vi "get_goal_filter.vi"(4 "Parameters":T2={"Stimulus"={"Type"=enum."Off", "Phase"=0.0, "Amplitude"=[], "Injection point"=enum."Total pose", "Closed loop"=FALSE, "Offset"=[], "Tip -> world"=FALSE, "Frequency"=0.0, "Length"=0.0}, "Goal Filter A"={"Speedup max"=0.0, "Speedup thresh"=0.0, "Speedup nonlin"=0.0, "Filters"=[]}, "Mode controls"={"Hold"=FALSE, "Cancellation"=FALSE, "Goal filter"=FALSE, "Trigger"=FALSE}, "Manipulator type"=enum."Current piezo", "Manipulator calibration"={"Tool offsets"=[[0.0, 0.0, 36200.0]], "Handle light calibration"=[], "Base pivots"=[], "Output pivots"=[], "Length center"=0.0, "Workspace height"=[], "Workspace diameter"=[0.0, 0.0, 36200.0], "Stack travel"=400.0, "Saturation pos"=375.0, "Inverse filters"=[], "Strut length"=0.0}, "Network"={"Remote Host"="", "Send Status"=FALSE, "Send Port"=0, "Recv Commands"=FALSE, "Recv Port"=0}, "Goal Filter B"={"Speedup max"=0.0, "Speedup thresh"=0.0, "Speedup nonlin"=0.0, "Filters"=[]}, "Cancellation"={"KP"={"XY"=0.0, "Rxy"=0.0, "Z"=0.0, "Rz"=0.0}, "KI"=0.0, "KD"={"XY"=0.0, "Rxy"=0.0, "Z"=0.0, "Rz"=0.0}, "Max vel"=20.0, "Max acc"=0.001, "Int error limit"=3.0, "RCM gain"=0.0, "Bypass"=FALSE, "Degraded gain"=0.0}, "Transition time"=0.0, "Estimation"={"Link"={"Measure noise"=[], "Process noise"=[], "Alt process noise"=[], "Alt turnoff cycles"=20, "Innovation limit"=[], "Residue threshold"=0.0, "Enable"=FALSE}, "Handle"={"Measure noise"=[], "Process noise"=[], "State limits"=[], "Innovation limit"=[], "Prediction Lookahead"=0.0, "Enable"=FALSE}}} {"Transition time" format="%_3f"; "Cancellation"."Degraded gain" min=0 max=1 step=0.1 format="%#_3p"; "Cancellation"."RCM gain" min=0 max=1 step=0.1 format="%#_3p"; "Cancellation"."KD"."Rz" min=-1 max=1 step=0.01 format="%#_3p"; "Cancellation"."KD"."Rxy" min=-1 max=1 step=0.01 format="%#_3p"; "Cancellation"."KD"."Z" min=-1 max=1 step=0.01 format="%#_3p"; "Cancellation"."KD"."XY" min=-1 max=1 step=0.01 format="%#_3p"; "Cancellation"."KI" min=0 max=1 step=0.01 format="%#_3p"; "Cancellation"."KP"."Rz" min=-1 max=1 step=0.01 format="%#_3p"; "Cancellation"."KP"."Rxy" min=-1 max=1 step=0.01 format="%#_3p"; "Cancellation"."KP"."Z" min=-1 max=1 step=0.01 format="%#_3p"; "Cancellation"."KP"."XY" min=-1 max=1 step=0.01 format="%#_3p"; "Cancellation"."Max acc" format="%#_3p"; "Goal Filter B"."Filters"."V limit range" format="%_3p"; "Goal Filter B"."Filters"."V limit" format="%_3p"; "Goal Filter B"."Filters"."Upper Q" format="%_3f"; "Goal Filter B"."Filters"."Upper Fc" format="%_3p"; "Goal Filter B"."Filters"."Lower Q" format="%_3f"; "Goal Filter B"."Filters"."Scale factor" format="%_3f"; "Goal Filter B"."Filters"."Lower Fc" format="%_3p"; "Goal Filter B"."Speedup nonlin" format="%_3p"; "Goal Filter B"."Speedup thresh" format="%_3p"; "Goal Filter B"."Speedup max" format="%_3p"; "Manipulator calibration"."Strut length" format="%#_4p"; "Manipulator calibration"."Saturation pos" format="%#.1f"; "Manipulator calibration"."Stack travel" format="%#.1f"; "Manipulator calibration"."Length center" format="%#_4p"; "Manipulator calibration"."Output pivots" format="%#_6f"; "Manipulator calibration"."Base pivots" format="%#_6f"; "Manipulator calibration"."Handle light calibration" format="%#.1f"; "Goal Filter A"."Filters"."V limit range" format="%_3p"; "Goal Filter A"."Filters"."V limit" format="%_3p"; "Goal Filter A"."Filters"."Upper Q" format="%_3f"; "Goal Filter A"."Filters"."Upper Fc" format="%_3p"; "Goal Filter A"."Filters"."Lower Q" format="%_3f"; "Goal Filter A"."Filters"."Scale factor" format="%_3f"; "Goal Filter A"."Filters"."Lower Fc" format="%_3p"; "Goal Filter A"."Speedup nonlin" format="%_3p"; "Goal Filter A"."Speedup thresh" format="%_3p"; "Goal Filter A"."Speedup max" format="%_3p"; "Stimulus"."Length" min=0.0 max=100.0 step=100.0 format="%#_4p"; "Stimulus"."Frequency" min=0.0 step=100.0 format="%#_4g"; "Stimulus"."Offset" format="%#_3p"; "Stimulus"."Amplitude" format="%#_3p"; "Stimulus"."Phase" min=-180.0 max=360.0 step=100.0 format="%#.2f"}, 5 "Sampling frequency":sgl=1.0 format="%0.2f") -> (1 "Goal loop params":T1={"Speedup max"=0.08, "Speedup thresh"=0.606, "Speedup nonlin"=3.0, "Filters"=[]} {"Filters"."V limit range" format="%_3p"; "Filters"."V limit" format="%_3p"; "Filters"."Upper Q" format="%_3f"; "Filters"."Upper Fc" format="%_3p"; "Filters"."Lower Q" format="%_3f"; "Filters"."Scale factor" format="%_3f"; "Filters"."Lower Fc" format="%_3p"; "Speedup nonlin" format="%_3p"; "Speedup thresh" format="%_3p"; "Speedup max" format="%_3p"})   [LabVIEW 2014]
uses:
  testing/Micron params.ctl
  testing/stimulus.ctl
  testing/injection_point.ctl
  goal_loop_parms.ctl
  testing/mode_conrols.ctl
  testing/manipulator_cal.ctl
  asap/labview/testing/probe_calibration.ctl
  host/network_params.ctl
  cancellation/sq_control_params.ctl
  cancellation/decoupled_gain.ctl
  cancellation/estimation_controls.ctl
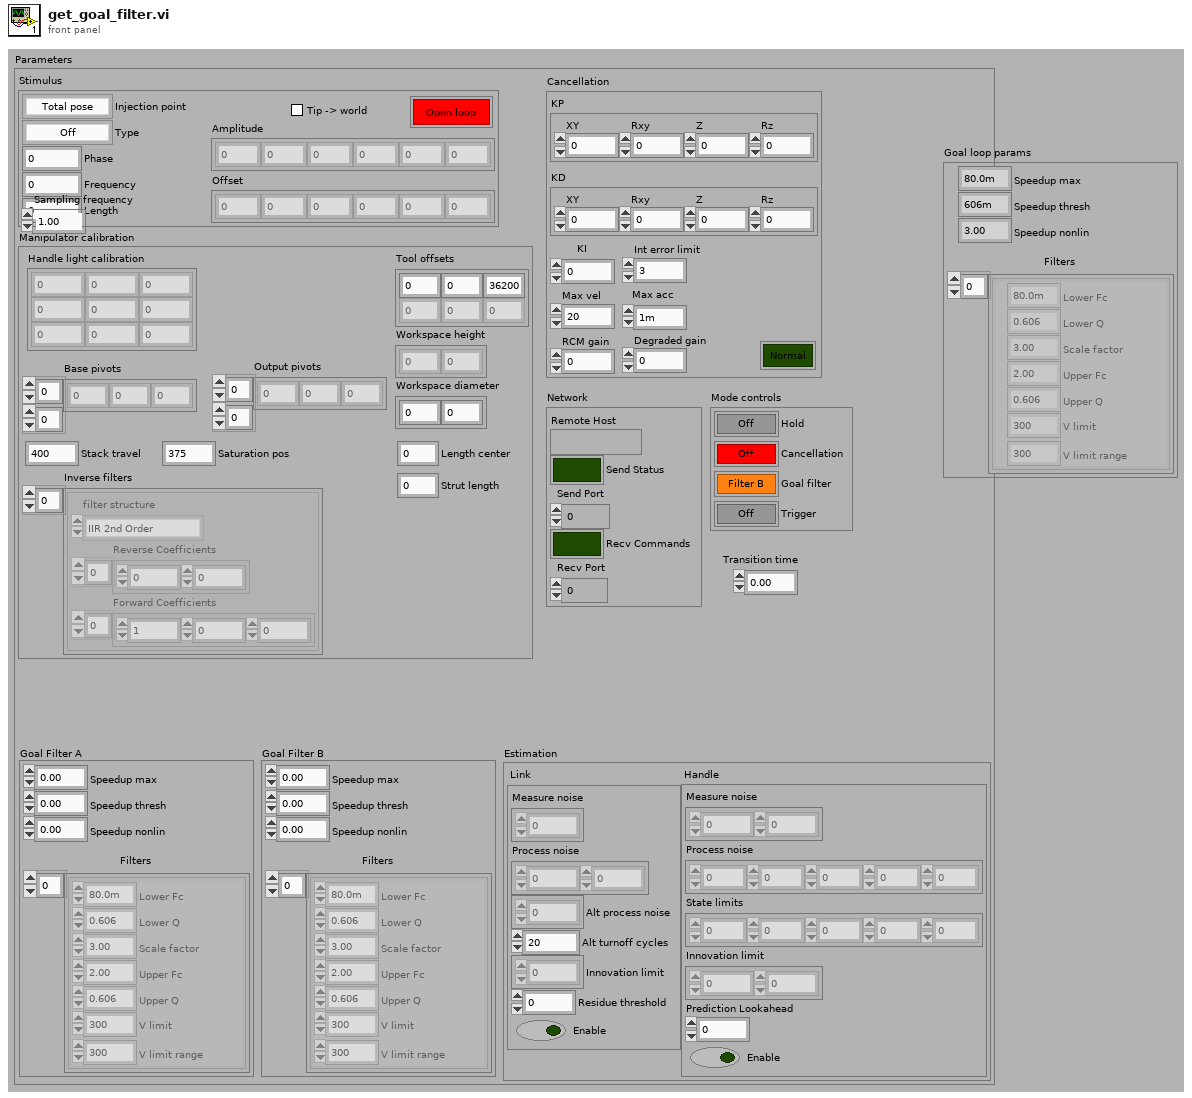
[diagram p1: front panel]
types:
  T1 = typedef "goal_loop_parms.ctl" = cluster{"Speedup max":sgl, "Speedup thresh":sgl, "Speedup nonlin":sgl, "Filters":cluster{"Lower Fc":sgl, "Lower Q":sgl, "Scale factor":sgl, "Upper Fc":sgl, "Upper Q":sgl, "V limit":sgl, "V limit range":sgl}[]}
  T2 = typedef "Micron params.ctl" = cluster{"Stimulus":T3, "Goal Filter A":T1, "Mode controls":T5, "Manipulator type":enum16{"Current piezo", "Voltage piezo"}, "Manipulator calibration":T6, "Network":T8, "Goal Filter B":T1, "Cancellation":T9, "Transition time":sgl, "Estimation":T11}
  T3 = typedef "stimulus.ctl" = cluster{"Type":enum16{"Off", "Step", "Sine", "Triangle", "Arbitrary"}, "Phase":dbl, "Amplitude":sgl[], "Injection point":T4, "Closed loop":bool, "Offset":sgl[], "Tip -> world":bool, "Frequency":dbl, "Length":dbl}
  T4 = typedef "injection_point.ctl" = enum16{"Total pose", "V limiter", "Goal ", "Link position", "KF link position", "Inverse kin", "Link goal", "Link error", "Controller", "Output", "Drive", "Light"}
  T5 = typedef "mode_conrols.ctl" = cluster{"Hold":bool, "Cancellation":bool, "Goal filter":bool, "Trigger":bool}
  T6 = typedef "manipulator_cal.ctl" = cluster{"Tool offsets":sgl[][], "Handle light calibration":T7, "Base pivots":sgl[][], "Output pivots":sgl[][], "Length center":sgl, "Workspace height":sgl[], "Workspace diameter":sgl[], "Stack travel":sgl, "Saturation pos":sgl, "Inverse filters":cluster{"filter structure":enum32{"IIR 2nd Order", "IIR 4th Order"}, "Reverse Coefficients":dbl[], "Forward Coefficients":dbl[]}[], "Strut length":sgl}
  T7 = typedef "probe_calibration.ctl" = sgl[][]
  T8 = typedef "network_params.ctl" = cluster{"Remote Host":string, "Send Status":bool, "Send Port":u16, "Recv Commands":bool, "Recv Port":u16}
  T9 = typedef "sq_control_params.ctl" = cluster{"KP":T10, "KI":sgl, "KD":T10, "Max vel":sgl, "Max acc":sgl, "Int error limit":sgl, "RCM gain":sgl, "Bypass":bool, "Degraded gain":sgl}
  T10 = typedef "decoupled_gain.ctl" = cluster{"XY":sgl, "Rxy":sgl, "Z":sgl, "Rz":sgl}
  T11 = typedef "estimation_controls.ctl" = cluster{"Link":cluster{"Measure noise":dbl[], "Process noise":dbl[], "Alt process noise":dbl[], "Alt turnoff cycles":i32, "Innovation limit":dbl[], "Residue threshold":dbl, "Enable":bool}, "Handle":cluster{"Measure noise":dbl[], "Process noise":dbl[], "State limits":dbl[], "Innovation limit":dbl[], "Prediction Lookahead":sgl, "Enable":bool}}
  T12 = cluster{"Lower Fc":sgl, "Lower Q":sgl, "Scale factor":sgl, "Upper Fc":sgl, "Upper Q":sgl, "V limit":sgl, "V limit range":sgl}[]
  T13 = cluster{"[0]":sgl, "[1]":sgl, "[2]":sgl, "[3]":sgl, "[4]":sgl, "[5]":sgl, "[6]":sgl}
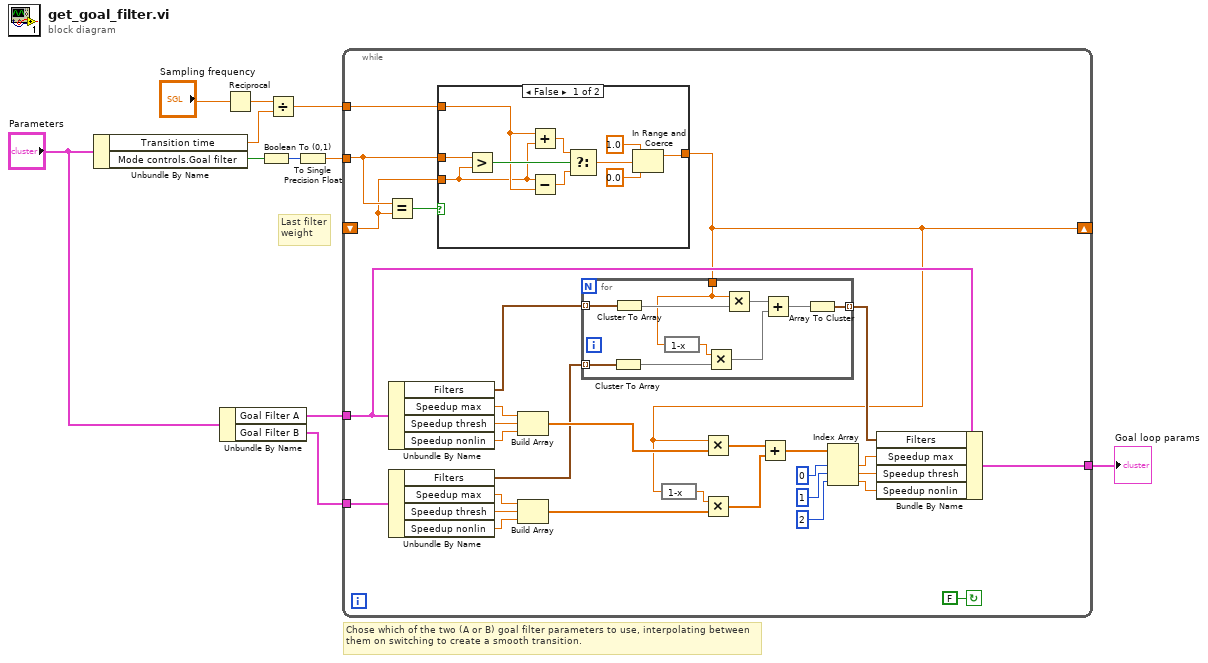
[diagram p0: block diagram]
diagram:
  # "Last filter\nweight"
  # "Chose which of the two (A or B) goal filter parameters to use, interpolating between them on switching to create a smooth transition."
  n1 = Unbundle By Name("Parameters") -> ("Transition time"=w6:sgl, "Mode controls.Goal filter"=w11:bool)
  n2 = Unbundle By Name("Parameters") -> ("Goal Filter A"=w3:T1, "Goal Filter B"=w2:T1)
  n3 = Reciprocal(x="Sampling frequency") -> (1/x=w7:sgl)
  n4 = Boolean To (0,1)(Boolean=w11) -> (0, 1=w10:i16)
  n5 = Divide(x=w7, y=w6) -> (x/y=w5:sgl)
  n6 = To Single Precision Float(number=w10) -> (single precision float=w9:sgl)
  n7 = while {
    tunnel: w9 -> [w38]
    shift-right: [w14] -> _
    shift-left: _ -> [w37]
    tunnel: w5 -> [w39]
    tunnel: w3 -> [w41]
    tunnel: w2 -> [w13]
    tunnel: [w12] -> w1
    stop <- FALSE continue-if-true
    n8 = Equal?(x=w38, y=w37) -> (x = y?=w36:bool)
    n9 = Unbundle By Name(w41) -> ("Filters"=w17:T12, "Speedup max"=w32:sgl, "Speedup thresh"=w31:sgl, "Speedup nonlin"=w30:sgl)
    n10 = Unbundle By Name(w13) -> ("Filters"=w16:T12, "Speedup max"=w27:sgl, "Speedup thresh"=w28:sgl, "Speedup nonlin"=w29:sgl)
    n11 = case shown="False" w36 {
      tunnel: w39 -> [w58 _]
      tunnel: w38 -> [w54 _]
      tunnel: w37 -> [w52 w62]
      tunnel: [w53 w62] -> w14
      frame False {
        n12 = Greater?(x=w54, y=w52) -> (0:w61:bool)
        n13 = Add(x=w58, y=w52) -> (x+y=w60:sgl)
        n14 = Subtract(x=w52, y=w58) -> (x-y=w59:sgl)
        n15 = Select(t=w60, s=w61, f=w59) -> (s? t:f=w57:sgl)
        n16 = In Range and Coerce(upper limit=sgl 1.0, x=w57, lower limit=sgl 0.0) -> (coerced(x)=w53:sgl)  [unwired: 1 out]
      }
      frame True {
      }
    }
    n17 = Build Array(w32, w31, w30) -> (w26:sgl[])
    n18 = Build Array(w27, w28, w29) -> (w25:sgl[])
    n19 = for {
      tunnel: [w45] -> w15 mode=indexing
      tunnel: w14 -> [w44]
      tunnel: w17 -> [w43] mode=indexing
      tunnel: w16 -> [w42] mode=indexing
      n20 = Cluster To Array(cluster=w42) -> (array=w49:sgl[])
      n21 = Cluster To Array(cluster=w43) -> (array=w51:sgl[])
      n22 = expression code="1-x"(w44) -> (w50:sgl)
      n23 = Multiply(x=w50, y=w49) -> (x*y=w47:sgl[])
      n24 = Multiply(x=w44, y=w51) -> (x*y=w48:sgl[])
      n25 = Add(x=w48, y=w47) -> (x+y=w46:sgl[])
      n26 = Array To Cluster(array=w46) -> (cluster=w45:T13)
    }
    n27 = expression code="1-x"(w14) -> (w33:sgl)
    n28 = Multiply(x=w14, y=w26) -> (x*y=w34:sgl[])
    n29 = Multiply(x=w33, y=w25) -> (x*y=w35:sgl[])
    n30 = Add(x=w34, y=w35) -> (x+y=w24:sgl[])
    n31 = Index Array(array=w24, index #1=0 ("index"), index #2=1 ("index"), index #3=2 ("index")) -> (element #1=w20:sgl, element #2=w19:sgl, element #3=w18:sgl)
    n32 = Bundle By Name(cluster=w41, "Filters"=w15, "Speedup max"=w20, "Speedup thresh"=w19, "Speedup nonlin"=w18) -> (w12:T1)
  }
  "Goal loop params" <- w1
